vi "Update Documentation.vi"(8 "error in":errorcluster, 10 "Documentation":T1, 11 "VI Map":T2) -> (0 "error out":errorcluster)   [LabVIEW 2021, in "Plugin Generator.lvlib"]
uses:
  Plugin Generator.lvlib
  <vilib>/Utility/traverseref.llb/TRef TravTarget.ctl
  <vilib>/Utility/traverseref.llb/VI Scripting - Traverse.lvlib
  <vilib>/CIF Foundation/CIF LabVIEW Scripting/LV Scripting/LV Scripting Utilities.lvlib
  <vilib>/CIF Foundation/CIF LabVIEW Scripting/LV Scripting/Typedef/Errors.ctl
  <vilib>/CIF Foundation/CIF LabVIEW Scripting/LV Scripting/Typedef/VI Map.ctl
  Typedef/Documentation Info.ctl
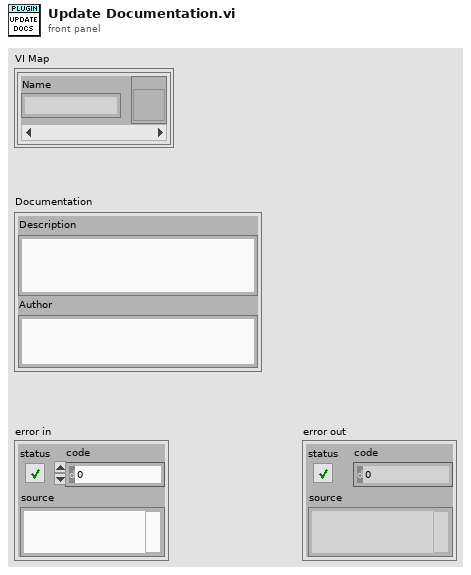
[diagram p1: front panel]
types:
  T1 = typedef "Plugin Generator.lvlib/Documentation Info.ctl" = cluster{"Description":string, "Author":string}
  T2 = typedef "LV Scripting Utilities.lvlib/VI Map.ctl" = map{string, refnum<vi>}
  T3 = typedef "Errors.ctl" = enum16{"Missing Version Changes", "Item not found"}
  T4 = typedef "TRef TravTarget.ctl" = enum16{"FP", "BD", "Other"}
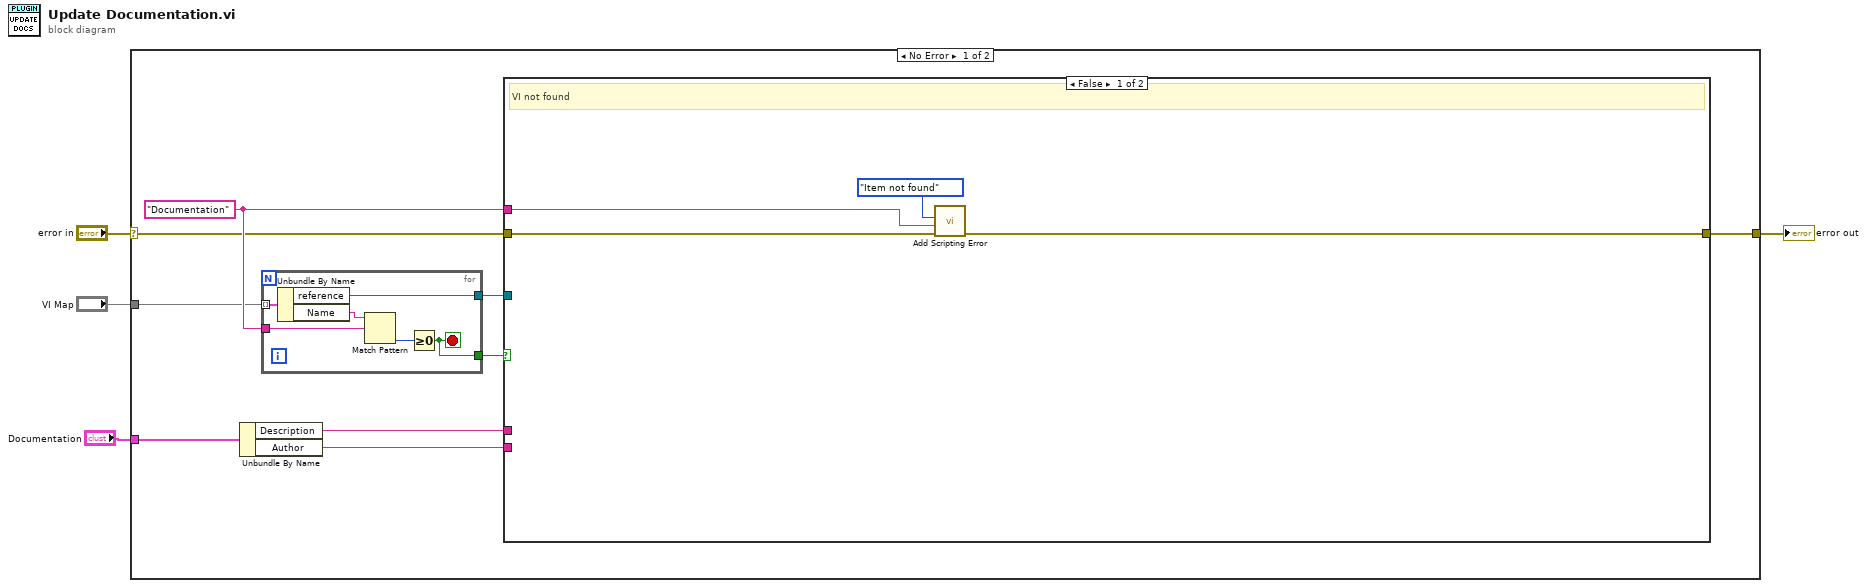
[diagram p0: block diagram]
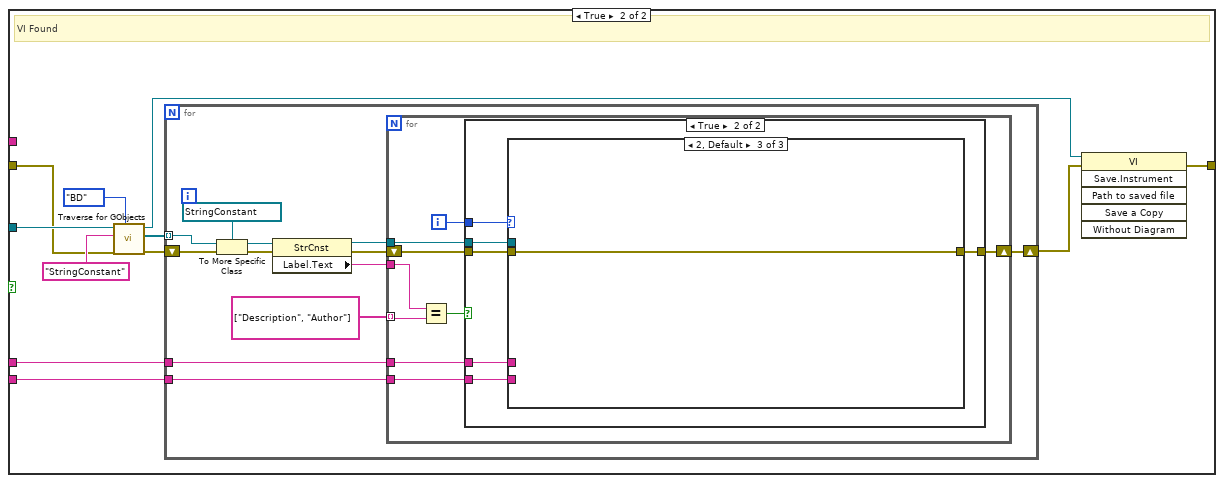
[diagram p2: hidden frame]
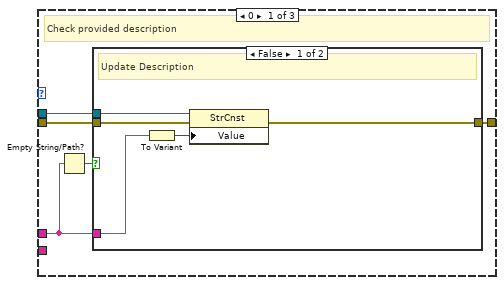
[diagram p4: hidden frame]
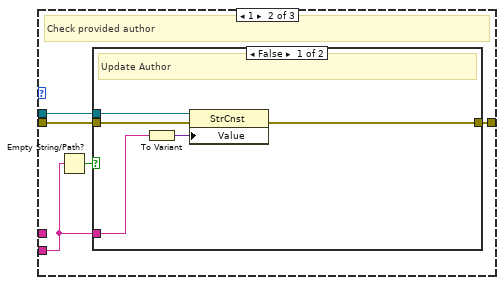
[diagram p6: hidden frame]
diagram:
  n1 = case shown="No Error" "error in" {
    selector: "error in" -> [w9 w86]
    tunnel: "VI Map" -> [w10 _]
    tunnel: [w8 w86] -> w2
    tunnel: "Documentation" -> [w7 _]
    frame No Error {
      w12 = "Documentation" ("Search Pattern")
      n2 = Unbundle By Name(w7) -> ("Description"=w6:string, "Author"=w5:string)
      n3 = for {
        tunnel: w10 -> [w19] mode=indexing
        tunnel: w12 -> [w18]
        tunnel: [w15] -> w13
        tunnel: [w14] -> w11
        stop <- w15 stop-if-true
        n4 = Unbundle By Name(w19) -> ("reference"=w14:refnum<vi>, "Name"=w16:string)
        n5 = Match Pattern(string=w16, regular expression=w18) -> (offset past match=w17:i32)  [unwired: 1 in, 3 out]
        n6 = Greater Or Equal To 0?(x=w17) -> (x >= 0?=w15:bool)
      }
      n7 = case shown="False" w13 {
        tunnel: w9 -> [w22 w25]
        tunnel: w12 -> [w20 _]
        tunnel: [w21 w27] -> w8
        tunnel: w5 -> [_ w24]
        tunnel: w6 -> [_ w31]
        tunnel: w11 -> [_ w26]
        frame False {
          # "VI not found"
          n8 = call <vilib>:"Add Scripting Error.vi"("error in (no error)"=w22, "String to Append"=w20, "Error"=Errors."Item not found") -> ("error out"=w21:errorcluster)  [unwired: 8 in]
        }
        frame True {
          # "VI Found"
          n9 = call <vilib>:"Traverse for GObjects.vi"("Traverse Target"=TRef_TravTarget."BD", "error in (no error)"=w25, "Class Name"="StringConstant", "VI Refnum"=w26) -> ("error out"=w30:errorcluster, "References"=w32:refnum<vi>[], "dup VI Refnum"=w29:refnum<vi>)  [unwired: 4 in, 1 out]
          n10 = for {
            tunnel: w32 -> [w46] mode=indexing
            tunnel: w24 -> [w39]
            shift-right: [w41] -> w28
            shift-left: w30 -> [w37]
            tunnel: w31 -> [w35]
            n11 = To More Specific Class(target class=refnum<vi> refnum ("x"), reference=w46, error in=w37) -> (specific class reference=w40:refnum<vi>, error out=w44:errorcluster)
            n12 = property class="StrCnst"(reference=w40, error in=w44) -> (reference out=w42:refnum<vi>, error out=w43:errorcluster, "Label.Text"=w38:string)
            n13 = for {
              tunnel: w42 -> [w54]
              tunnel: w39 -> [w52]
              tunnel: w38 -> [w49]
              shift-right: [w53] -> w41
              shift-left: w43 -> [w55]
              tunnel: string[] ["Description", "Author"] -> [w51] mode=indexing
              tunnel: w35 -> [w47]
              i -> [w48]
              n14 = Equal?(x=w49, y=w51) -> (x = y?=w50:bool)
              n15 = case shown="True" w50 {
                tunnel: w55 -> [w56 w60]
                tunnel: w54 -> [_ w62]
                tunnel: [w56 w61] -> w53
                tunnel: w52 -> [_ w57]
                tunnel: w48 -> [_ w59]
                tunnel: w47 -> [_ w58]
                frame False {
                }
                frame True {
                  n16 = case shown="2, Default" w59 {
                    tunnel: w62 -> [w67 w78 _]
                    tunnel: [w66 w77 w85] -> w61
                    tunnel: w60 -> [w65 w76 w85]
                    tunnel: w58 -> [w63 _ _]
                    tunnel: w57 -> [_ w74 _]
                    frame 0 {
                      # "Check provided description"
                      n17 = Empty String/Path?(string/path=w63) -> (empty?=w64:bool)
                      n18 = case shown="False" w64 {
                        tunnel: w67 -> [w69 _]
                        tunnel: [w71 w73] -> w66
                        tunnel: w65 -> [w68 w73]
                        tunnel: w63 -> [w70 _]
                        frame False {
                          # "Update Description"
                          n19 = To Variant(anything=w70) -> (Variant=w72:variant)
                          n20 = property class="StrCnst"(reference=w69, error in=w68, "Value"=w72) -> (error out=w71:errorcluster)  [unwired: 1 out]
                        }
                        frame True {
                          # "No update provided"
                        }
                      }
                    }
                    frame 1 {
                      # "Check provided author"
                      n21 = Empty String/Path?(string/path=w74) -> (empty?=w75:bool)
                      n22 = case shown="False" w75 {
                        tunnel: w78 -> [w80 _]
                        tunnel: [w82 w84] -> w77
                        tunnel: w76 -> [w79 w84]
                        tunnel: w74 -> [w81 _]
                        frame False {
                          # "Update Author"
                          n23 = To Variant(anything=w81) -> (Variant=w83:variant)
                          n24 = property class="StrCnst"(reference=w80, error in=w79, "Value"=w83) -> (error out=w82:errorcluster)  [unwired: 1 out]
                        }
                        frame True {
                          # "No update provided"
                        }
                      }
                    }
                    frame 2, Default {
                    }
                  }
                }
              }
            }
          }
          n25 = invoke class="VI" method="Save.Instrument"(reference=w29, error in=w28) -> (error out=w27:errorcluster)  [unwired: 4 in, 5 out]
        }
      }
    }
    frame Error {
    }
  }
  "error out" <- w2
